vi "onDataUpdate.vi"(7 "SenderName":string, 8 "error in":errorcluster, 9 "ObservableValue":variant, 10 "ObservableName":string, 11 "ObserverClass in":refnum<class "ObserverClass.lvclass">) -> (0 "error out":errorcluster, 1 "IsSender":bool, 3 "ObserverClass out":refnum<class "ObserverClass.lvclass">)   [LabVIEW 2025, in "ObserverClass.lvlib" / "ObserverClass.lvclass"]
doc: "Update Observable Data"
uses:
  ObserverClass.lvclass
  ObserverClass.lvclass/ObserverClass.ctl
  ObserverClass.lvlib
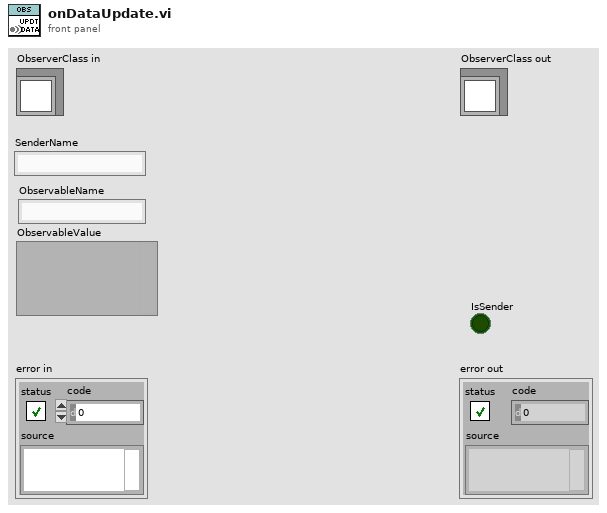
[diagram p1: front panel]
types:
  T1 = enum16{"Get", "Set", "Init", "Remove", "Destroy"}
  T2 = map{string, cluster{"ObserverEvent":refnum<user-event>, "ObserverNr":u64, "ObservableValue":variant}}
  T3 = map{string, cluster{"ObserverEvent":refnum<user-event>, "ObserverNr":u64, "Value":variant}}
  T4 = cluster{"ObserverEvent":refnum<user-event>, "ObserverNr":u64, "Value":variant}
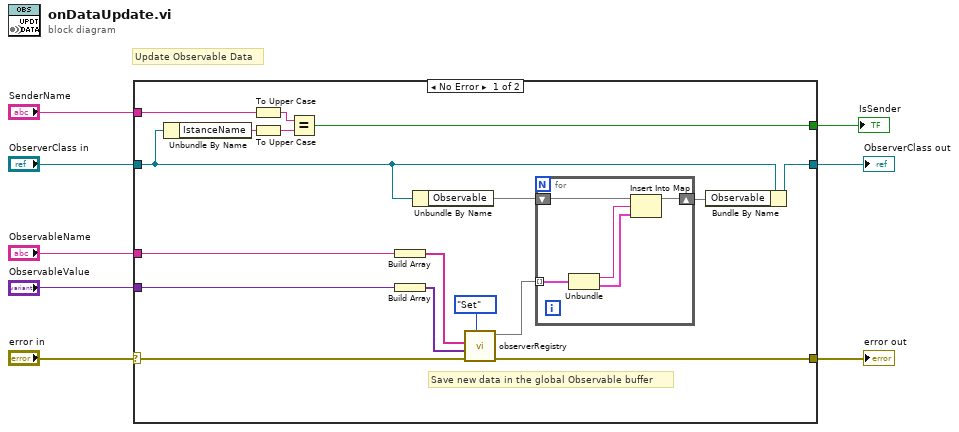
[diagram p0: block diagram]
diagram:
  # "Update Observable Data"
  n1 = case shown="No Error" "error in" {
    selector: "error in" -> [w23 w32]
    tunnel: [w24 w32] -> w7
    tunnel: [w25 w31] -> w5
    tunnel: "ObserverClass in" -> [w22 w31]
    tunnel: "ObservableName" -> [w17 _]
    tunnel: "ObservableValue" -> [w16 _]
    tunnel: "SenderName" -> [w18 _]
    tunnel: [w9 _] -> w1
    frame No Error {
      # "Save new data in the global Observable buffer"
      n2 = Unbundle By Name(w22) -> ("IstanceName"=w20:string)
      n3 = To Upper Case(1:w18) -> (0:w19:string)
      n4 = To Upper Case(1:w20) -> (0:w21:string)
      n5 = Equal?(x=w19, y=w21) -> (x = y?=w9:bool)
      n6 = Build Array(w17) -> (w14:string[])
      n7 = Build Array(w16) -> (w13:variant[])
      n8 = Unbundle By Name(w22) -> ("Observable"=w11:T2)
      n9 = call "observerRegistry.vi"("Action"=T1."Set", "error in"=w23, "ObservableValue"=w13, "ObservableName"=w14) -> ("error out"=w24:errorcluster, "Observable out"=w12:T3)  [unwired: 5 in, 1 out]
      n10 = for {
        tunnel: w12 -> [w30] mode=indexing
        shift-right: [w28] -> w10
        shift-left: w11 -> [w29]
        n11 = Unbundle(w30) -> ("Name"=w27:string, "ObserverInfo"=w26:T4)
        n12 = Insert Into Map(map in=w29, key=w27, value=w26) -> (map out=w28:T2)  [unwired: 2 out]
      }
      n13 = Bundle By Name(cluster=w22, "Observable"=w10) -> (w25:refnum<class "ObserverClass.lvclass">)
    }
    frame Error {
    }
  }
  "error out" <- w7
  "ObserverClass out" <- w5
  "IsSender" <- w1
